vi "VHM-disconnect.vi"(8 "error in (no error)":errorcluster, 11 "VHM-VNA_Hardware_Manager in":refnum<class "VHM-VNA_Hardware_Manager.lvclass">) -> (0 "error out":errorcluster, 3 "VHM-VNA_Hardware_Manager out":refnum<class "VHM-VNA_Hardware_Manager.lvclass">)   [LabVIEW 2020, in "VHM-VNA_Hardware_Manager.lvlib" / "VHM-VNA_Hardware_Manager.lvclass"]
uses:
  VHM-VNA_Hardware_Manager.lvclass
  VHM-VNA_Hardware_Manager.lvclass/VHM-VNA_Hardware_Manager.ctl
  classes/vna-drivers/liteVNA/VD-LV-LiteVNA.lvclass
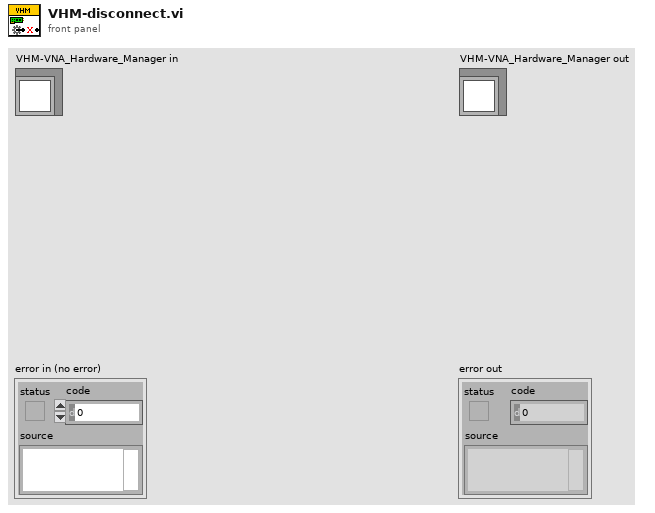
[diagram p1: front panel]
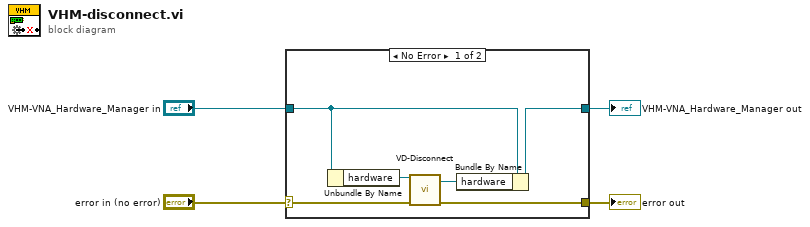
[diagram p0: block diagram]
diagram:
  n1 = case shown="No Error" "error in (no error)" {
    selector: "error in (no error)" -> [w6 w12]
    tunnel: [w5 w12] -> w3
    tunnel: [w10 w11] -> w1
    tunnel: "VHM-VNA_Hardware_Manager in" -> [w9 w11]
    frame No Error {
      n2 = Unbundle By Name(w9) -> ("hardware"=w8:refnum<class "VD-LV-LiteVNA.lvclass">)
      n3 = call-dynamic "VD-Disconnect.vi"("error in (no error)"=w6, "VD-LV-LiteVNA in"=w8) -> ("error out"=w5:errorcluster, "VD-LV-LiteVNA out"=w7:refnum<class "VD-LV-LiteVNA.lvclass">)  [unwired: 8 in]
      n4 = Bundle By Name(cluster=w9, "hardware"=w7) -> (w10:refnum<class "VHM-VNA_Hardware_Manager.lvclass">)
    }
    frame Error {
    }
  }
  "error out" <- w3
  "VHM-VNA_Hardware_Manager out" <- w1
